vi "Get TextDocument Refnum.vi"(8 "error in (no error)":errorcluster, 11 "ooWriter in":refnum<class "ooWriter.lvclass">) -> (0 "error out":errorcluster, 2 "TextDocument":refnum<k24>, 3 "ooWriter out":refnum<class "ooWriter.lvclass">)   [LabVIEW 2009, in "ooWriter.lvclass"]
uses:
  ooWriter.lvclass
  C:/Projets/LAVAG/OpenOfficeRGT/AODL/DLLs/AODL.dll
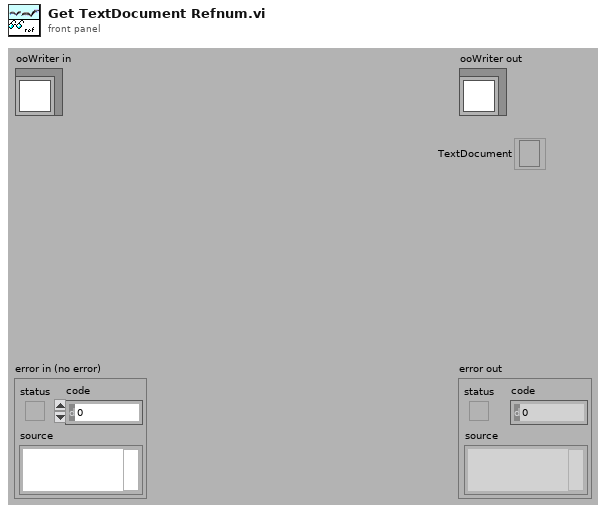
[diagram p1: front panel]
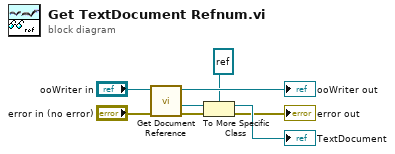
[diagram p0: block diagram]
diagram:
  n1 = call-dynamic "Get Document Reference.vi"("error in (no error)"="error in (no error)", "ooDocument in"="ooWriter in") -> ("error out"=w6:errorcluster, "Document"=w5:refnum<k24>, "ooDocument out"=→"ooWriter out":refnum<class "ooWriter.lvclass">)  [unwired: 7 in]
  n2 = To More Specific Class(target class=refnum<k24> refnum ("TextDocument"), reference=w5, error in=w6) -> (specific class reference=→"TextDocument":refnum<k24>, error out=→"error out":errorcluster)
